vi "fun draw.vi"() -> ()   [LabVIEW 2009]
uses:
  <vilib>/Utility/miscctls.llb/LVPoint32TypeDef.ctl
panel:
  in  "clear":bool
  in  "stop":bool
  out "XY Graph":cluster{"Horizontal":i32, "Vertical":i32}[](graph)
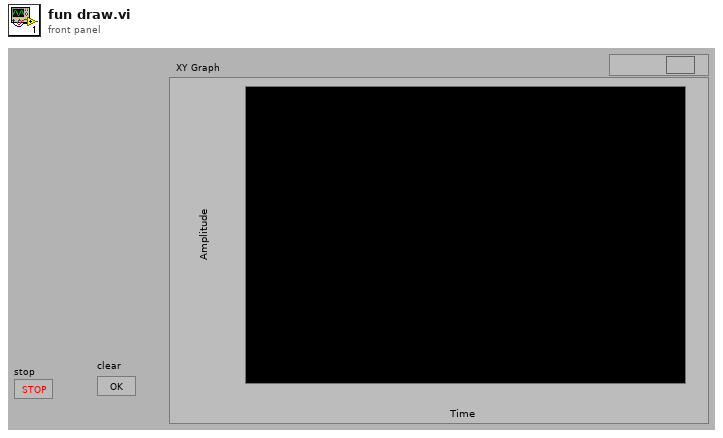
[diagram p1: front panel]
types:
  T1 = typedef "LVPoint32TypeDef.ctl" = cluster{"Horizontal":i32, "Vertical":i32}
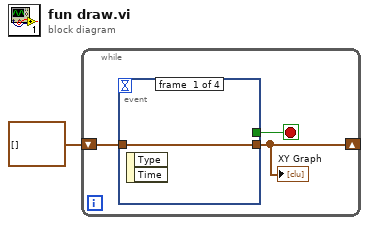
[diagram p0: block diagram]
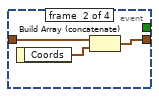
[diagram p2: hidden frame]
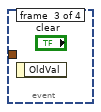
[diagram p3: hidden frame]
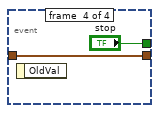
[diagram p4: hidden frame]
diagram:
  n1 = while {
    shift-right: [w2] -> _
    shift-left: T1[] [] -> [w3]
    stop <- w4 stop-if-true
    n2 = event shown="[2] \"clear\": Value Change" {
      selector: _ -> [_ _ _ _]
      dyn-events: _ -> [_ _ _ _]
      timeout: _ -> [_ _ _ _]
      tunnel: [_ _ _ "stop"] -> w4
      tunnel: w3 -> [w5 w8 _ w9]
      tunnel: [w5 w7 _ w9] -> w2
      event #0 {
        n3 = event-data() -> ()  [unwired: 1 in, 2 out]
      }
      event #1 {
        n4 = event-data() -> ("Coords"=w6:T1)  [unwired: 1 in]
        n5 = Build Array (concatenate)(w8, w6) -> (w7:T1[])
      }
      event #2 {
        n6 = event-data() -> ()  [unwired: 1 in, 1 out]
      }
      event #3 {
        n7 = event-data() -> ()  [unwired: 1 in, 1 out]
      }
    }
    "XY Graph" <- w2
  }
